vi "save processed data (XYplot).vi"(8 "error in (no error)":errorcluster, 10 "Processed data (XY plot)":cluster{dbl[], dbl[]}[](graph), 11 "Task in":refnum<class "Task.lvclass">) -> (0 "error out":errorcluster, 3 "Task out":refnum<class "Task.lvclass">)   [LabVIEW 2020, in "Tasks.lvlib" / "Task.lvclass"]
uses:
  Task.lvclass
  Task.lvclass/Task.ctl
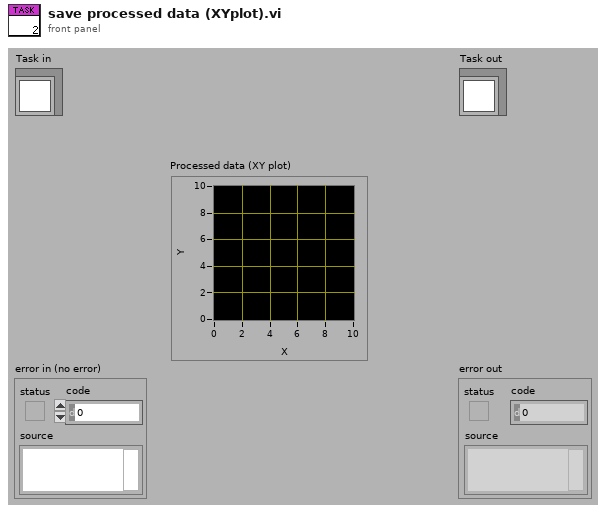
[diagram p1: front panel]
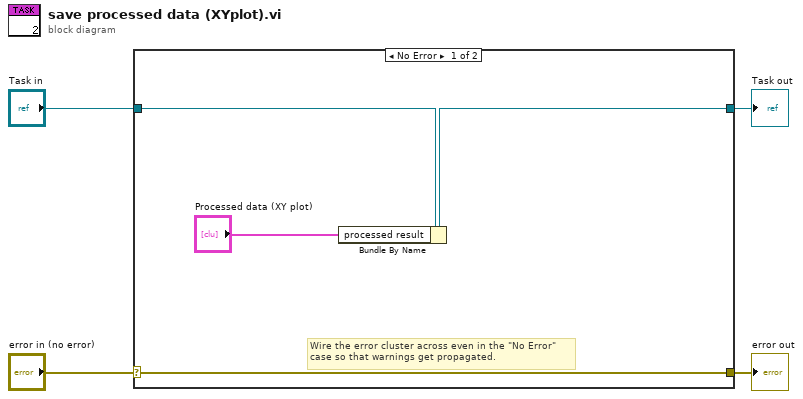
[diagram p0: block diagram]
diagram:
  n1 = case shown="No Error" "error in (no error)" {
    selector: "error in (no error)" -> [w8 w10]
    tunnel: [w8 w10] -> w3
    tunnel: [w5 w9] -> w1
    tunnel: "Task in" -> [w6 w9]
    frame No Error {
      # "Wire the error cluster across even in the \"No Error\"\ncase so that warnings get propagated."
      n2 = Bundle By Name(cluster=w6, "processed result"="Processed data (XY plot)") -> (w5:refnum<class "Task.lvclass">)
    }
    frame Error {
    }
  }
  "error out" <- w3
  "Task out" <- w1
